vi "xyyy plot.vi"(5 "Y column":i32, 7 "X column":i32, 8 "error in (no error)":errorcluster, 11 "file path (dialog if empty)":path[](array[path])) -> (0 "error out":errorcluster, 3 "output cluster":cluster{dbl[], dbl[]}[](array[cluster]))   [LabVIEW 2021]
uses:
  <vilib>/Utility/file.llb/Read Delimited Spreadsheet (DBL).vi
panel:
  # "Accept data in columns with Xs and Ys"
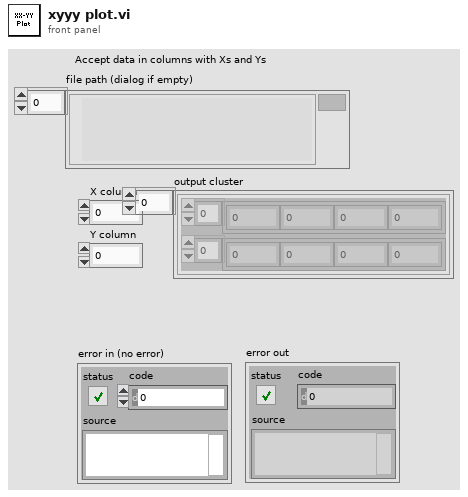
[diagram p1: front panel]
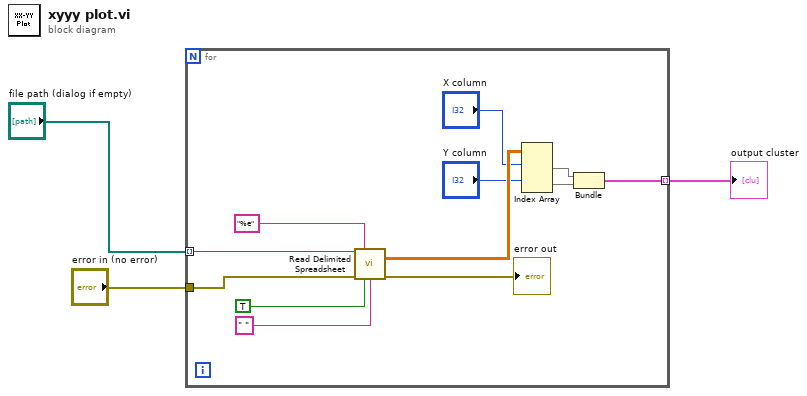
[diagram p0: block diagram]
diagram:
  n1 = for {
    tunnel: "error in (no error)" -> [w14]
    tunnel: [w8] -> w1 mode=indexing
    tunnel: "file path (dialog if empty)" -> [w4] mode=indexing
    n2 = call-poly <vilib>:"Read Delimited Spreadsheet.vi"("file path (dialog if empty)"=w4, "format (%.3f)"="%e", "error in (no error)"=w14, "transpose? (F)"=TRUE, "delimiter (\\t)"=" " ("delimiter (\\t)")) -> ("all rows"=w13:dbl[][], "error out"=→"error out":errorcluster)  [unwired: 5 in, 4 out]
    n3 = Index Array(array=w13, index (row) #1="X column", index (row) #2="Y column") -> (element #1=w10:dbl[], element #2=w9:dbl[])  [unwired: 2 in]
    n4 = Bundle("all rows"=w10, "all rows"=w9) -> (w8:cluster{"all rows":dbl[], "all rows":dbl[]})  [unwired: 1 in]
  }
  "output cluster" <- w1
